vi "Get_LEM_Response.vi"(6 "Frequency (Hz)":dbl, 8 "Cavity Pressure Magnitude":dbl, 9 "Cavity Pressure Phase":dbl, 10 "Fluid Properties":T1={"R"=8.31451, "Mair"=0.0289645, "T"=293.0, "Patmos"=101325.0, "gamma"=1.4}, 11 "SJ Data IN":T2) -> (0 "Phi":dbl, 1 "Phi*":dbl, 2 "Uo":dbl, 3 "U*":dbl, 4 "OmegaH":dbl)   [LabVIEW 2011]
uses:
  Controls/SJ_Data_Cluster.ctl
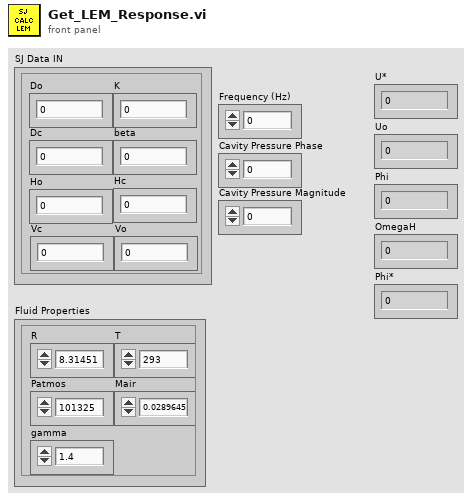
[diagram p1: front panel]
types:
  T1 = cluster{"R":dbl, "Mair":dbl, "T":dbl, "Patmos":dbl, "gamma":dbl}
  T2 = typedef "SJ_Data_Cluster.ctl" = cluster{"Do":dbl, "Dc":dbl, "Ho":dbl, "Hc":dbl, "K":dbl, "beta":dbl, "Vc":dbl, "Vo":dbl}
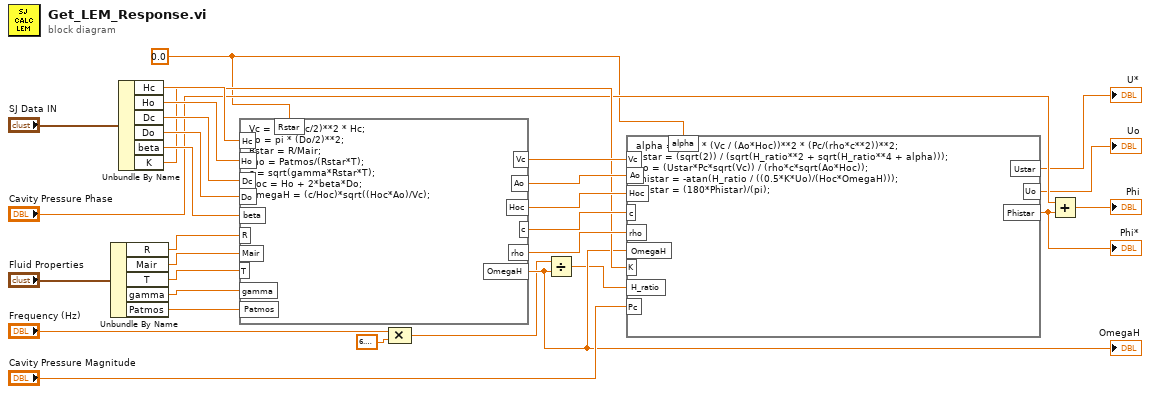
[diagram p0: block diagram]
diagram:
  w6 = 0.0 ("input variable")
  n1 = Unbundle By Name("Fluid Properties") -> ("R"=w25:dbl, "Mair"=w24:dbl, "T"=w23:dbl, "gamma"=w22:dbl, "Patmos"=w21:dbl)
  n2 = Unbundle By Name("SJ Data IN") -> ("Hc"=w30:dbl, "Ho"=w29:dbl, "Dc"=w28:dbl, "Do"=w27:dbl, "beta"=w14:dbl, "K"=w13:dbl)
  n3 = formula code="Vc = pi * (Dc/2)**2 * Hc; \nAo = pi * (Do/2)**2;\nRstar = R/Mair; \nrho = Patmos/(Rstar*T);\nc = sqrt(gamma*Rstar*T); \nHoc = Ho + 2*beta*Do; \nOmegaH = (c/Hoc)*sqrt((Hoc*Ao)/Vc);"("Do"=w27, "R"=w25, "Mair"=w24, "T"=w23, "gamma"=w22, "Ho"=w29, "Dc"=w28, "Hc"=w30, "Patmos"=w21, "beta"=w14, "Rstar"=w6) -> ("Vc"=w20:dbl, "Ao"=w19:dbl, "Hoc"=w18:dbl, "c"=w17:dbl, "rho"=w16:dbl, "OmegaH"=w3:dbl)
  "OmegaH" <- w3
  n4 = Compound Arithmetic op=MULTIPLY("Frequency (Hz)", 6.283185307179586) -> (w2:dbl)
  n5 = Divide(x=w2, y=w3) -> (x/y=w1:dbl)
  n6 = formula code="alpha = K**2 * (Vc / (Ao*Hoc))**2 * (Pc/(rho*c**2))**2;\nUstar = (sqrt(2)) / (sqrt(H_ratio**2 + sqrt(H_ratio**4 + alpha)));\nUo = (Ustar*Pc*sqrt(Vc)) / (rho*c*sqrt(Ao*Hoc));\nPhistar = -atan(H_ratio / ((0.5*K*Uo)/(Hoc*OmegaH)));\nPhistar = (180*Phistar)/(pi);"("c"=w17, "rho"=w16, "OmegaH"=w3, "K"=w13, "H_ratio"=w1, "Ao"=w19, "Hoc"=w18, "Vc"=w20, "Pc"="Cavity Pressure Magnitude", "alpha"=w6) -> ("Ustar"=→"U*":dbl, "Uo"=→"Uo":dbl, "Phistar"=w10:dbl)
  "Phi*" <- w10
  n7 = Add(x="Cavity Pressure Phase", y=w10) -> (x+y=→"Phi":dbl)
